vi "Multiple motor operation(Wheel mode).vi"() -> ()   [LabVIEW 2016]
uses:
  <instrlib>/Dynamixel Motor/Public/Motor Operation/Low Level/Baud Setting.ctl
  <instrlib>/Dynamixel Motor/Dynamixel Motor.lvlib
panel:
  in  "Goal Speed 2 (RPM)":dbl
  in  "Goal Speed 1 (RPM)":dbl
  in  "Motor 2 ID (0)":u8
  in  "Motor 1 ID (0)":u8
  in  "정지":bool
  in  "Baud rate (57600 bps)":T1=34 items=["1,000,000 bps"=1, "500,000 bps"=3, "400,000 bps"=4, "250,000 bps"=7, "200,000 bps"=9, "115200 bps"=16, "57600 bps"=34, "19200 bps"=103, "9600 bps"=207]
  in  "VISA resource name":refnum<visa-resource-name>
  # "Motor 1 Configuration"
  # "Motor 2 Configuration"
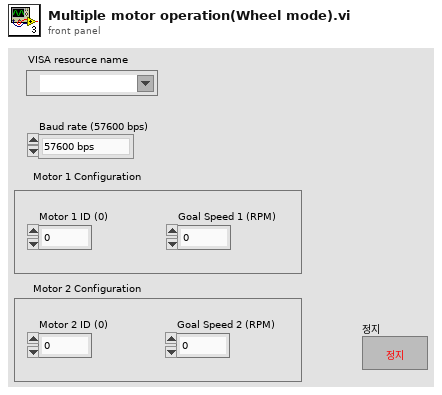
[diagram p1: front panel]
types:
  T1 = typedef "Dynamixel Motor.lvlib/Baud Setting.ctl" = u8
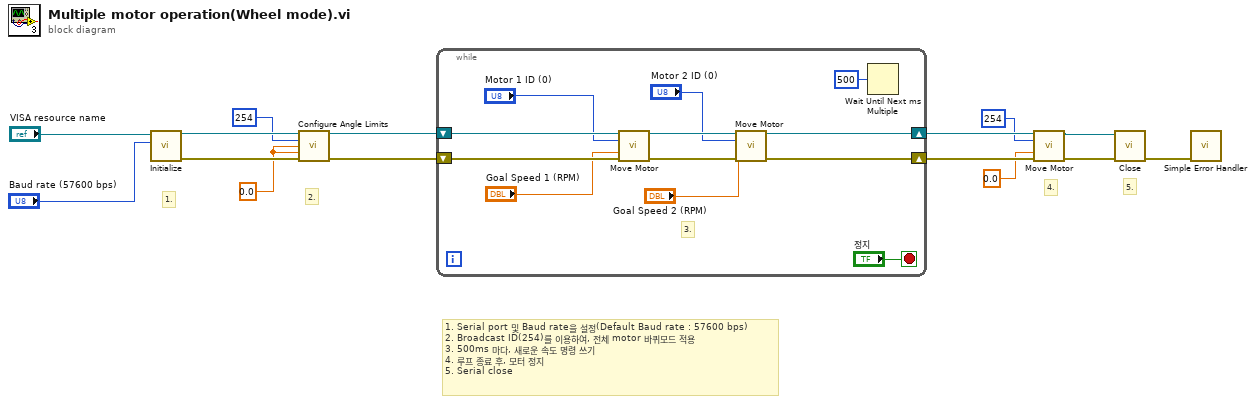
[diagram p0: block diagram]
diagram:
  w8 = 0.0 ("Clockwise Angle Limit (0 deg)")
  # "5."
  # "1. Serial port 및 Baud rate을 설정(Default Baud rate : 57600 bps)\n2. Broadcast ID(254)를 이용하여, 전체 motor 바퀴모드 적용\n3. 500ms 마다, 새로운 속도 명령 쓰기\n4. 루프 종료 후, 모터 정지\n5. Serial close"
  # "2."
  # "4."
  # "1."
  n1 = call <instrlib>:"Initialize.vi"("Baud rate (57600 bps)"="Baud rate (57600 bps)", "VISA resource name"="VISA resource name") -> ("error out"=w14:errorcluster, "VISA resource name out"=w15:refnum<visa-resource-name>)  [unwired: 8 in]
  n2 = call <instrlib>:"Configure Angle Limits.vi"("VISA resource name"=w15, "Motor ID (0)"=u8 254, "Clockwise Angle Limit (0 deg)"=w8, "Counter-Clockwise Angle Limit (300 deg)"=w8, "error in (no error)"=w14) -> ("VISA resource name out"=w10:refnum<visa-resource-name>, "error out"=w9:errorcluster)  [unwired: 9 in]
  n3 = while {
    shift-right: [w21] -> w5
    shift-left: w10 -> [w27]
    shift-right: [w20] -> w4
    shift-left: w9 -> [w26]
    stop <- "정지" stop-if-true
    # "3."
    n4 = call <instrlib>:"Move Motor.vi"("VISA resource name"=w27, "Motor ID (0)"="Motor 1 ID (0)", "Goal Speed (RPM)"="Goal Speed 1 (RPM)", "error in (no error)"=w26) -> ("VISA resource name out"=w23:refnum<visa-resource-name>, "error out"=w22:errorcluster)  [unwired: 10 in]
    n5 = call <instrlib>:"Move Motor.vi"("VISA resource name"=w23, "Motor ID (0)"="Motor 2 ID (0)", "Goal Speed (RPM)"="Goal Speed 2 (RPM)", "error in (no error)"=w22) -> ("VISA resource name out"=w21:refnum<visa-resource-name>, "error out"=w20:errorcluster)  [unwired: 10 in]
    n6 = Wait Until Next ms Multiple(millisecond multiple=u32 500 ("ms 배수")) -> ()  [unwired: 1 out]
  }
  n7 = call <instrlib>:"Move Motor.vi"("VISA resource name"=w5, "Motor ID (0)"=u8 254, "Goal Speed (RPM)"=0.0, "error in (no error)"=w4) -> ("VISA resource name out"=w3:refnum<visa-resource-name>, "error out"=w6:errorcluster)  [unwired: 10 in]
  n8 = call <instrlib>:"Close.vi"("error in (no error)"=w6, "VISA resource name"=w3) -> ("error out"=w13:errorcluster)  [unwired: 9 in]
  n9 = call <vilib>:"Simple Error Handler.vi"("error in (no error)"=w13) -> ()  [unwired: 4 in, 5 out]
